vi "Report Event.vi"(7 "Level (Info)":T1=enum."Info", 8 "error in (no error)":errorcluster, 9 "Message":string, 10 "Context":string, 11 "VolatusCore in":refnum<class "VolatusCore.lvclass">) -> (0 "error out":errorcluster, 3 "VolatusCore out":refnum<class "VolatusCore.lvclass">)   [LabVIEW 2020, in "Volatus.lvlib" / "VolatusCore.lvclass"]
uses:
  VolatusCore.lvclass
  VolatusCore.lvclass/VolatusCore.ctl
  Event API/EventAPI.lvclass
  Event Level.ctl
  Volatus.lvlib
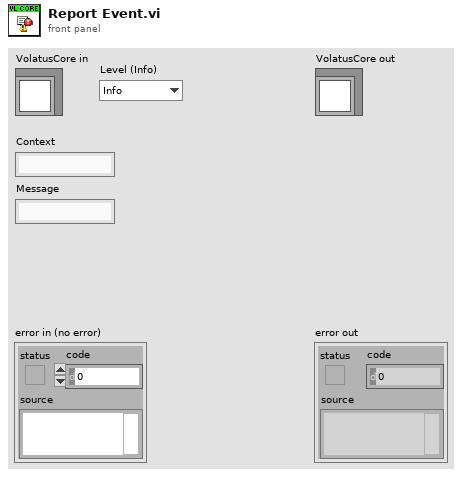
[diagram p1: front panel]
types:
  T1 = typedef "Volatus.lvlib/Event Level.ctl" = enum16{"Debug", "Info", "Warning", "Error"}
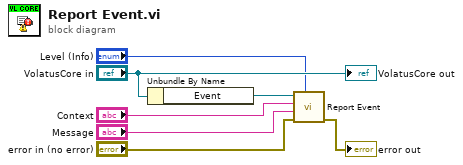
[diagram p0: block diagram]
diagram:
  n1 = Unbundle By Name("VolatusCore in") -> ("Event"=w6:refnum<class "EventAPI.lvclass">)
  n2 = call "Report Event.vi"("Level (Info)"="Level (Info)", "error in (no error)"="error in (no error)", "Message"="Message", "Context"="Context", "Event API in"=w6) -> ("error out"=→"error out":errorcluster)  [unwired: 5 in, 1 out]
  "VolatusCore out" <- "VolatusCore in"
